vi "Calc - RhoH20.vi"(11 "TFFT":dbl) -> (3 "RhoH20":dbl)   [LabVIEW 2018, in "Controller (Host).lvlib"]
uses:
  Controller (Host).lvlib
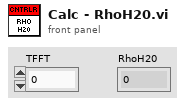
[diagram p1: front panel]
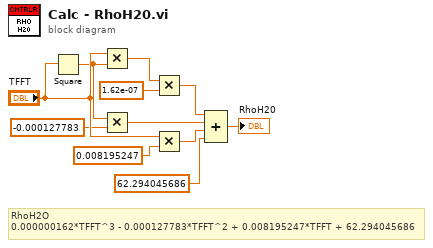
[diagram p0: block diagram]
diagram:
  # "RhoH2O\n0.000000162*TFFT^3 - 0.000127783*TFFT^2 + 0.008195247*TFFT + 62.294045686"
  n1 = Square(x="TFFT") -> (x^2=w2:dbl)
  n2 = Multiply(x="TFFT", y=w2) -> (x*y=w1:dbl)
  n3 = Multiply(x=w2, y=-0.000127783) -> (x*y=w4:dbl)
  n4 = Multiply(x=w1, y=1.62e-07) -> (x*y=w3:dbl)
  n5 = Multiply(x="TFFT", y=0.008195247) -> (x*y=w5:dbl)
  n6 = Compound Arithmetic op=ADD(w3, w4, w5, 62.294045686 ("value")) -> (→"RhoH20":dbl)
